vi "Set Self Attributes.vi"(10 "Self Attributes":T1, 11 "Sender in":refnum<class "Sender.lvclass">) -> (3 "Sender out":refnum<class "Sender.lvclass">)   [LabVIEW 2020, in "jettl.lvlib" / "Sender.lvlib" / "Sender.lvclass"]
uses:
  Sender.lvclass
  Msg/Msg.lvclass
  Actor/Implemented Msgs.ctl
  Actor/Actor.lvlib
  Actor/Attributes.ctl
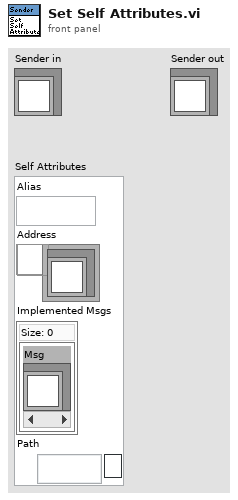
[diagram p1: front panel]
types:
  T1 = typedef "jettl.lvlib/Actor.lvlib/Attributes.ctl" = cluster{"Alias":string, "Address":refnum<user-event>, "Implemented Msgs":T2, "Path":path}
  T2 = typedef "jettl.lvlib/Actor.lvlib/Implemented Msgs.ctl" = set{refnum<class "Msg.lvclass">}
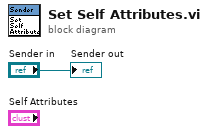
[diagram p0: block diagram]
diagram:
  "Sender out" <- "Sender in"
